vi "RSNRPZ Get Scope Measurements Pulse Power.vi"(8 "error in (no error)":errorcluster, 10 "Channel (1)":i32=1, 11 "VISA session":refnum<visa-resource-name> caption="VISA resource name") -> (0 "error out":errorcluster, 1 "Average":dbl format="%^.3e", 3 "dup VISA session":refnum<visa-resource-name> caption="VISA resource name", 4 "Min Peak":dbl format="%^.3e", 5 "Max Peak":dbl format="%^.3e")   [LabVIEW 2010]
doc: "This VI returns the average power, the minimum level and the maximum level of the analysed trace in Watt.\n\nNote:\n1) This VI is only available for NRP-Z81.\n\nRemote-control command(s):\nSENS:TRAC:MEAS:POW:AVG?\nSENS:TRAC:MEAS:POW:MIN?\nSENS:TRAC:MEAS:POW:MAX?"
uses:
  rsnrpz_32.dll
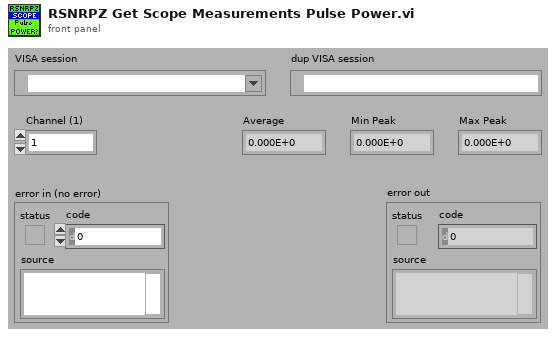
[diagram p1: front panel]
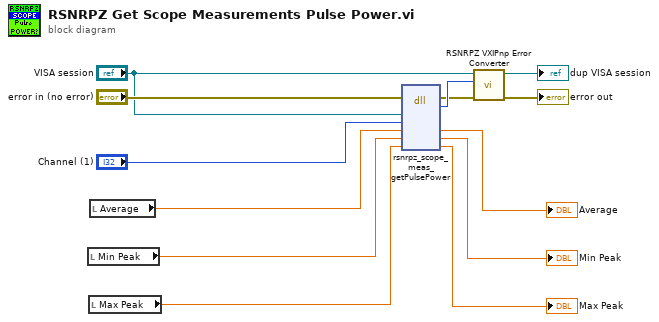
[diagram p0: block diagram]
diagram:
  n1 = local read "Min Peak"() -> (w9:dbl)
  n2 = local read "Max Peak"() -> (w7:dbl)
  n3 = local read "Average"() -> (w11:dbl)
  n4 = dll-call lib="rsnrpz_32.dll" fn="rsnrpz_scope_meas_getPulsePower"(error in="error in (no error)", "Instrument Handle"="VISA session", "Channel"="Channel (1)", "Average"=w11, "Min Peak"=w9, "Max Peak"=w7) -> (error out=w5:errorcluster, "Status"=w13:i32, "Average"=→"Average":dbl, "Min Peak"=→"Min Peak":dbl, "Max Peak"=→"Max Peak":dbl)  [unwired: 4 in, 1 out]
  n5 = call <instrlib>:"RSNRPZ VXIPnp Error Converter.vi"("error in"=w5, "VXIPnp error code"=w13, "VISA session"="VISA session") -> ("error out"=→"error out":errorcluster, "dup VISA session"=→"dup VISA session":refnum<visa-resource-name>)  [unwired: 7 in]
